vi "MQM Data Transfer All.vi"() -> ()   [LabVIEW 2023]
uses:
  Typedefs/ZI_Frontpanel_All.ctl
  Typedefs/PPMS_Status.ctl
  Typedefs/Rotator_Status.ctl
panel:
  in  "Rotator":T1
  in  "PPMS":T2
  in  "ZI MFLI":T3 {"Lockin 4 Demod 0"."frequency (Hz)" format="%#_6p"; "Lockin 4 Demod 0"."X(V)" format="%#_6p"; "Lockin 4 Demod 0"."R(V)" format="%#_6p"; "Lockin 3 Demod 0"."X(V)" format="%#_6p"; "Lockin 3 Demod 0"."R(V)" format="%#_6p"; "Lockin 2 Demod 0"."X(V)" format="%#_6p"; "Lockin 2 Demod 0"."R(V)" format="%#_6p"; "Lockin 1 Demod 0"."X(V)" format="%#_6p"; "Lockin 1 Demod 0"."R(V)" format="%#_6p"}
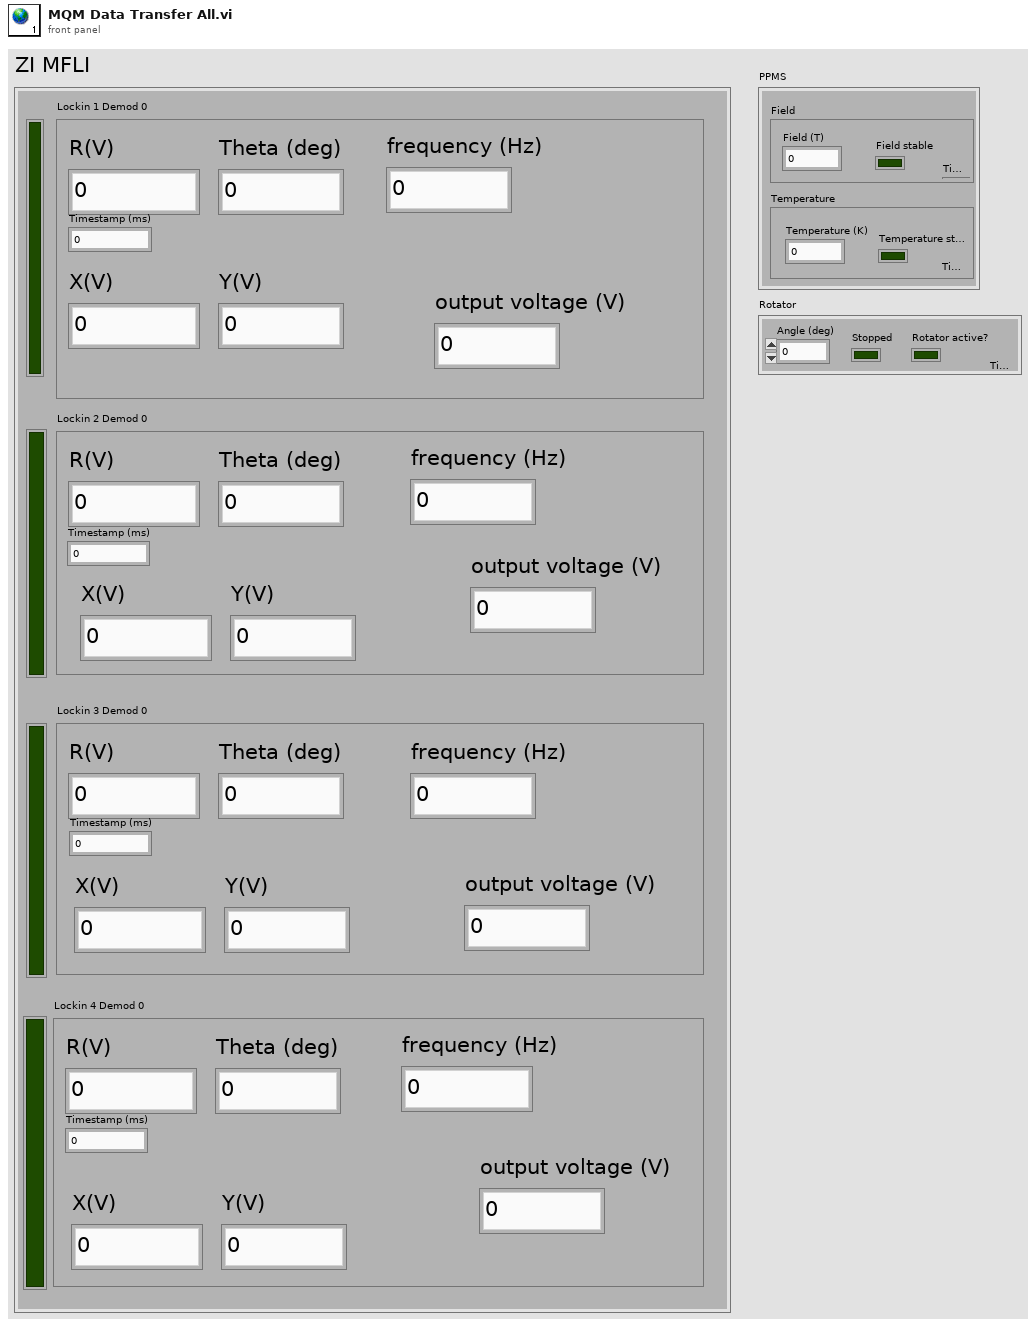
[diagram p1: front panel]
types:
  T1 = typedef "Rotator_Status.ctl" = cluster{"Angle (deg)":dbl, "Stopped":bool, "Rotator active?":bool, "Timestamp (ms)":u32}
  T2 = typedef "PPMS_Status.ctl" = cluster{"Field":cluster{"Field (T)":dbl, "Field stable":bool, "Timestamp (ms)":u32}, "Temperature":cluster{"Temperature (K)":dbl, "Temperature stable":bool, "Timestamp (ms)":u32}}
  T3 = typedef "ZI_Frontpanel_All.ctl" = cluster{"Lockin 1 Demod 0":cluster{"R(V)":dbl, "Theta (deg)":dbl, "Timestamp (ms)":u32, "X(V)":dbl, "Y(V)":dbl, "frequency (Hz)":dbl, "output voltage (V)":dbl}, "Lockin 2 Demod 0":cluster{"R(V)":dbl, "Theta (deg)":dbl, "Timestamp (ms)":u32, "X(V)":dbl, "Y(V)":dbl, "frequency (Hz)":dbl, "output voltage (V)":dbl}, "Lockin 3 Demod 0":cluster{"R(V)":dbl, "Theta (deg)":dbl, "Timestamp (ms)":u32, "X(V)":dbl, "Y(V)":dbl, "frequency (Hz)":dbl, "output voltage (V)":dbl}, "Lockin 4 Demod 0":cluster{"R(V)":dbl, "Theta (deg)":dbl, "Timestamp (ms)":u32, "X(V)":dbl, "Y(V)":dbl, "frequency (Hz)":dbl, "output voltage (V)":dbl}, "LI1 active":bool, "LI2 active":bool, "LI3 active":bool, "LI4 active":bool}
diagram:
